vi "Pick Object by Data.vi"() -> ()   [LabVIEW 2020]
panel:
  in  "O":refnum<class>[](array[class])
  in  "Conditional Object Array":refnum<class>[](array[class])
  in  "Object B Array":refnum<class>[](array[class])
  in  "Object A Array":refnum<class>[](array[class])
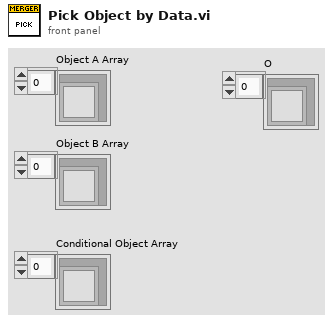
[diagram p1: front panel]
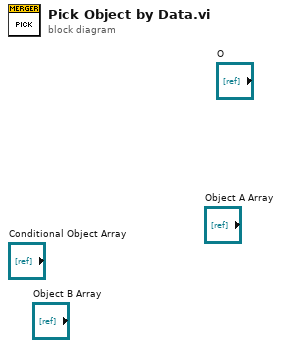
[diagram p0: block diagram]
diagram:
